vi "Check_Conn-s_bet-n_Displ_in_Track_Group-1.vi"(4 "error IN":errorcluster, 6 "[IN] # of Unconne\ncted Problem points":i32, 7 "[IN] Clusters for Re\nconstructed Tracks":T1) -> (0 "error OUT":errorcluster, 2 "[OUT] # of Unconne\ncted Problem points":i32, 3 "[OUT] Clusters for Re\nconstructed Tracks":T1)   [LabVIEW 2013]
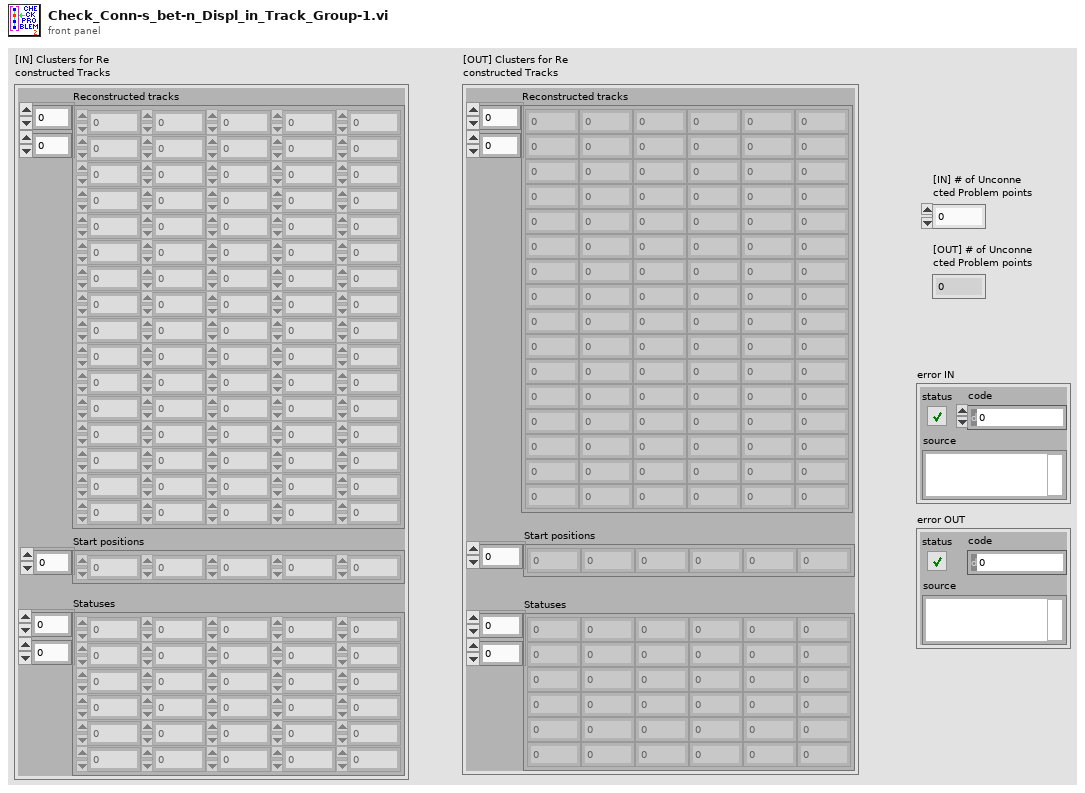
[diagram p1: front panel]
types:
  T1 = cluster{"Reconstructed tracks":dbl[][], "Start positions":i32[], "Statuses":i16[][]}
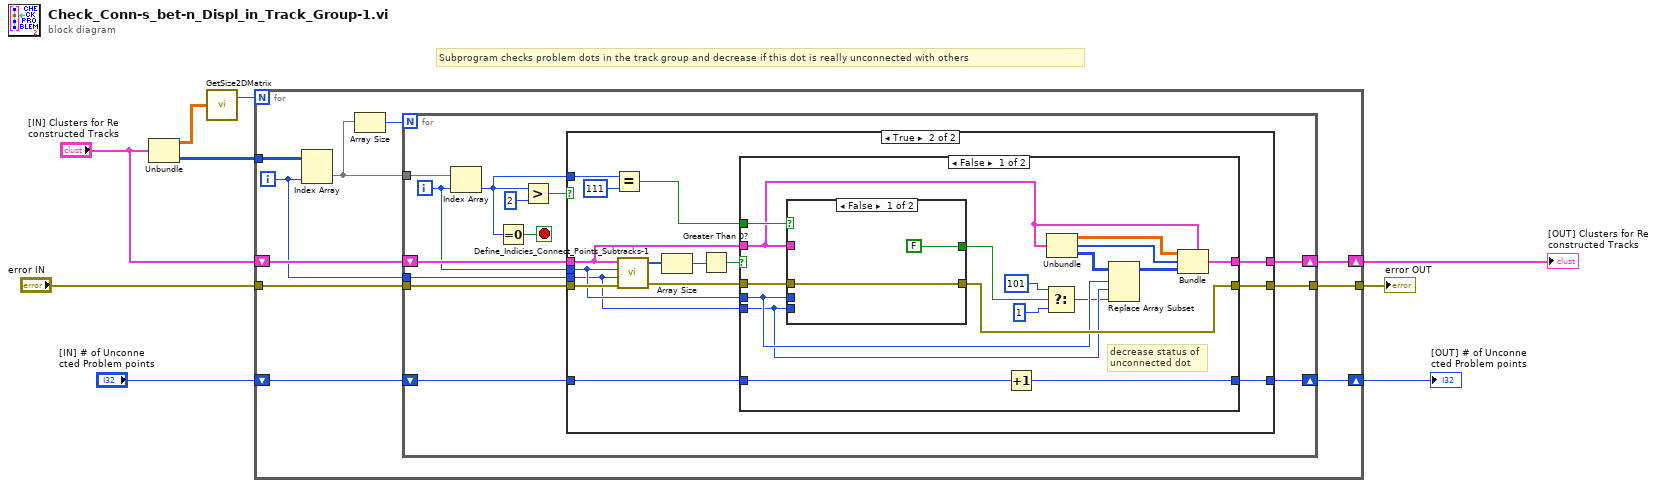
[diagram p0: block diagram]
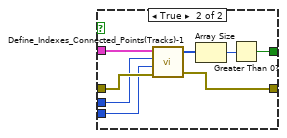
[diagram p3: hidden frame]
diagram:
  # "Subprogram checks problem dots in the track group and decrease if this dot is really unconnected with others"
  n1 = Unbundle("[IN] Clusters for Re\nconstructed Tracks") -> ("Reconstructed tracks"=w5:dbl[][], "Statuses"=w3:i16[][])  [unwired: 1 out]
  n2 = call "GetSize2DMatrix.vi"("Array IN (2D)"=w5) -> ("# Cols"=w4:i32)  [unwired: 1 out]
  n3 = for {
    N: w4 -> [_]
    tunnel: w3 -> [w19]
    shift-right: [w13] -> w1
    shift-left: "[IN] Clusters for Re\nconstructed Tracks" -> [w16]
    tunnel: "error IN" -> [w14]
    shift-right: [w11] -> w6
    shift-left: "[IN] # of Unconne\ncted Problem points" -> [w12]
    tunnel: [w10] -> w7
    i -> [w15]
    n4 = Index Array(array=w19, index (col)=w15) -> (element=w17:i16[])  [unwired: 1 in]
    n5 = Array Size(array=w17) -> (size(s)=w18:i32)
    n6 = for {
      N: w18 -> [_]
      tunnel: w17 -> [w32]
      shift-right: [w24] -> w13
      shift-left: w16 -> [w28]
      tunnel: w15 -> [w26]
      tunnel: w14 -> [w25]
      shift-right: [w22] -> w11
      shift-left: w12 -> [w23]
      tunnel: [w21] -> w10
      i -> [w27]
      stop <- w31 stop-if-true
      n7 = Index Array(array=w32, index=w27) -> (element=w20:i16)
      n8 = Equal To 0?(x=w20) -> (x = 0?=w31:bool)
      n9 = Greater?(x=w20, y=i16 2) -> (0:w29:bool)
      n10 = case shown="True" w29 {
        tunnel: w28 -> [w35 w43]
        tunnel: w27 -> [_ w42]
        tunnel: w26 -> [_ w41]
        tunnel: w25 -> [w34 w44]
        tunnel: [w35 w48] -> w24
        tunnel: w23 -> [w33 w47]
        tunnel: [w33 w46] -> w22
        tunnel: [w34 w45] -> w21
        tunnel: w20 -> [_ w38]
        frame False {
        }
        frame True {
          n11 = Equal?(x=w38, y=i16 111) -> (x = y?=w36:bool)
          n12 = call "Define_Indicies_Connect_Points_Subtracks-1.vi"("error IN"=w44, "[IN] Index of track with\n(problem displacement)"=w41, "[IN] Index of problem\ndisplacement inside track"=w42, "[IN] Track group"=w43) -> ("error OUT"=w39:errorcluster, "[OUT] Index of connected\ntracks with problem dot"=w40:i32[])  [unwired: 1 out]
          n13 = Array Size(array=w40) -> (size(s)=w50:i32)
          n14 = Greater Than 0?(x=w50) -> (x > 0?=w49:bool)
          n15 = case shown="False" w49 {
            tunnel: w43 -> [w61 w80]
            tunnel: [w60 w80] -> w48
            tunnel: w47 -> [w52 w78]
            tunnel: [w51 w78] -> w46
            tunnel: w42 -> [w55 _]
            tunnel: w41 -> [w54 _]
            tunnel: w39 -> [w66 w79]
            tunnel: [w59 w79] -> w45
            tunnel: w36 -> [w67 _]
            frame False {
              # "decrease status of \nunconnected dot"
              n16 = case shown="False" w67 {
                tunnel: w61 -> [_ w77]
                tunnel: w66 -> [w68 w76]
                tunnel: w55 -> [_ w75]
                tunnel: w54 -> [_ w74]
                tunnel: [FALSE w71] -> w58
                tunnel: [w68 w70] -> w59
                frame False {
                }
                frame True {
                  n17 = call "Define_Indexes_Connected_Points(Tracks)-1.vi"("error IN"=w76, "[IN] Index of track with\n(problem displacement)"=w74, "[IN]Index of problem\ndisplacement inside track"=w75, "[IN] Track group"=w77) -> ("error OUT"=w70:errorcluster, "[OUT] Index of connected\ntracks with problem dot"=w72:i32[])  [unwired: 1 out]
                  n18 = Array Size(array=w72) -> (size(s)=w73:i32)
                  n19 = Greater Than 0?(x=w73) -> (x > 0?=w71:bool)
                }
              }
              n20 = Increment(x=w52) -> (x+1=w51:i32)
              n21 = Select(t=i16 101 ("new element/subarray"), s=w58, f=i16 1 ("new element/subarray")) -> (s? t:f=w53:i16)
              n22 = Unbundle(w61) -> ("Reconstructed tracks"=w63:dbl[][], "Start positions"=w64:i32[], "Statuses"=w62:i16[][])
              n23 = Replace Array Subset(array=w62, new element=w53, index (row)=w55, index (col)=w54) -> (w65:i16[][])
              n24 = Bundle(cluster=w61, "Reconstructed tracks"=w63, "Start positions"=w64, "Statuses"=w65) -> (w60:T1)
            }
            frame True {
            }
          }
        }
      }
    }
  }
  "error OUT" <- w7
  "[OUT] # of Unconne\ncted Problem points" <- w6
  "[OUT] Clusters for Re\nconstructed Tracks" <- w1
